vi "stopBuildWorker.vi"(8 "error in (no error)":errorcluster, 11 "BuildWorker in":refnum<class "BuildWorker.lvclass">) -> (0 "error out":errorcluster, 3 "BuildWorker out":refnum<class "BuildWorker.lvclass">)   [LabVIEW 2017, in "BuildWorker Interface.lvlib" / "BuildWorker.lvclass"]
uses:
  BuildWorker.lvclass
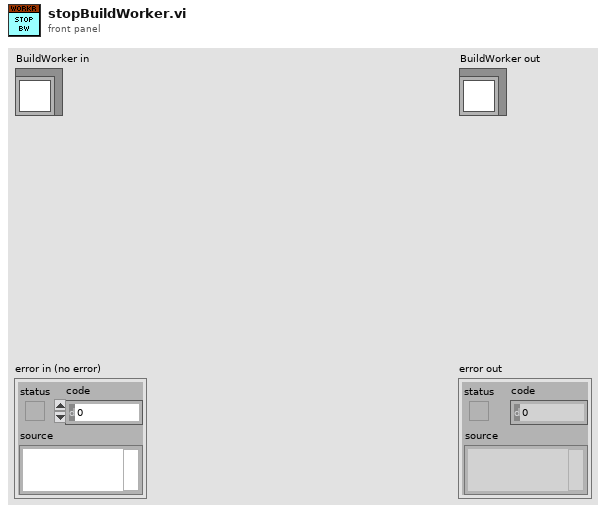
[diagram p1: front panel]
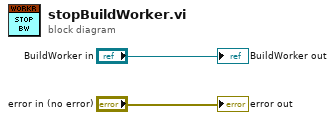
[diagram p0: block diagram]
diagram:
  "error out" <- "error in (no error)"
  "BuildWorker out" <- "BuildWorker in"
